vi "未命名 1.vi"() -> ()   [LabVIEW 2012]
uses:
  <vilib>/ptbypt/NI_PtbyPt.lvlib
panel:
  in  "输入":dbl
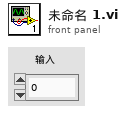
[diagram p1: front panel]
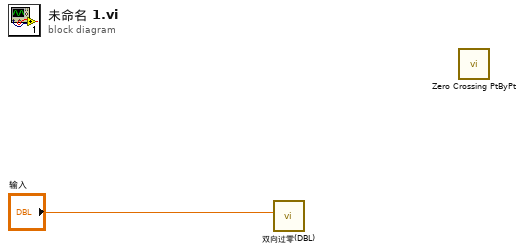
[diagram p0: block diagram]
diagram:
  n1 = call "双向过零(DBL).vi"("输入"="输入") -> ()  [unwired: 7 in, 1 out]
  n2 = call <vilib>:"Zero Crossing PtByPt.vi"() -> ()  [unwired: 3 in, 1 out]
